vi "Main v0.5.vi"() -> ()   [LabVIEW 2017]
doc: "v0.5:\n\n- Added Reject to Manual Mode\n- Send reject pallet cluster during manual mode\n- Run continuous manual happens only when no error has occured"
uses:
  Controls/Main Tabs.ctl
  Controls/Auto.ctl
  RT/Controls/Auto Delays.ctl
  RT/Controls/Auto Times.ctl
  <userlib>/SESL Controls/refresh ES.ctl
  Controls/UI Data.ctl
  support/Message Queue/Enqueue Message (Single).vi
  <vilib>/Utility/error.llb/Error Cluster From Error Code.vi
  <vilib>/ErrorRing/Error Ring.xnode
  support/Message Queue/Message Queue.lvlib
  support/User Event - Stop/User Event - Stop.lvlib
panel:
  out "Date-Time":string caption="Dip-Tube Assembly Automation (HMI) v0.5"
  out "Main Tab":T1
  in  "Autocycle":T2
  in  "Manual":bool
  in  "Parameters":bool
  in  "Maintenance":bool
  in  "Save Para":bool
  in  "Home Para":bool
  in  "ParaTab":T3(tab)
  in  "StopperRearDelay":dbl format="%#.2f"
  in  "StopperFrontDelay":dbl format="%#.2f"
  in  "MaxAlarms":dbl caption="Max Alarms in 1 Minute" format="%#.2f"
  in  "MaxConsecutive":dbl caption="Max Consecutive Alarms" format="%#.2f"
  in  "Gate Close Delay":dbl format="%#.2f"
  in  "Gate Open Delay":dbl format="%#.2f"
  in  "BF Off Delay":dbl format="%#.2f"
  in  "BF On Delay":dbl format="%#.2f"
  in  "DelayAfterReject":dbl format="%#.2f"
  in  "MeasurementTime":dbl format="%#.2f"
  in  "DelayAfterMesFront":dbl format="%#.2f"
  in  "DelayAfterCut":dbl format="%#.2f"
  in  "DelayAfterCutClamp":dbl format="%#.2f"
  in  "DelayAfterInsClamp":dbl format="%#.2f"
  in  "DelayToClose":dbl format="%#.2f"
  in  "DelayToOpen":dbl format="%#.2f"
  in  "DelayAfterInsertion":dbl format="%#.2f"
  in  "DelayBeforeInsertion":dbl format="%#.2f"
  in  "AgitatorUpTime":dbl format="%#.2f"
  in  "AgitatorDownTime":dbl format="%#.2f"
  in  "Reject Pallets":T4
  in  "Enable Reject?":bool
  in  "Toggle Motor":bool
  in  "Continuous?":T5
  in  "Enable Measure?":bool
  in  "Enable Index?":bool
  in  "Enable PF?":bool
  in  "Auto Delays":T6={"Agitator Delays"=[400], "TF Delays"=[500], "Insertion Delays"=[100, 500], "Cutting Delays"=[150, 500, 100], "PF Delays"=[100], "Measur. Delays"=[500], "Reject Delays"=[500]}
  in  "Enable Cutting?":bool
  in  "Enable Insertion?":bool
  in  "Run Manual":bool
  in  "Enable TF?":bool
  in  "Home Manual":bool
  out "Status":T8
  out "Measurements":T9 {"Height 1" format="%#.2f"; "Height 2" format="%#.2f"; "Height 3" format="%#.2f"; "Height 4" format="%#.2f"}
  out "OutputCount":u32
  in  "All IO":bool
  in  "Stats":bool
  in  "Home AC":bool
  out "Status":string
  out "Count":dbl format="%06.0f"
  out "Count 3":dbl caption="Cycle Time" format="%0.2f"
  out "Count 2":dbl caption="Rejects" format="%06.0f"
  in  "Statuses":string[][](table)
  in  "Exit":bool
  # "Vision Harmony Dip-Tube Assembly Automation"
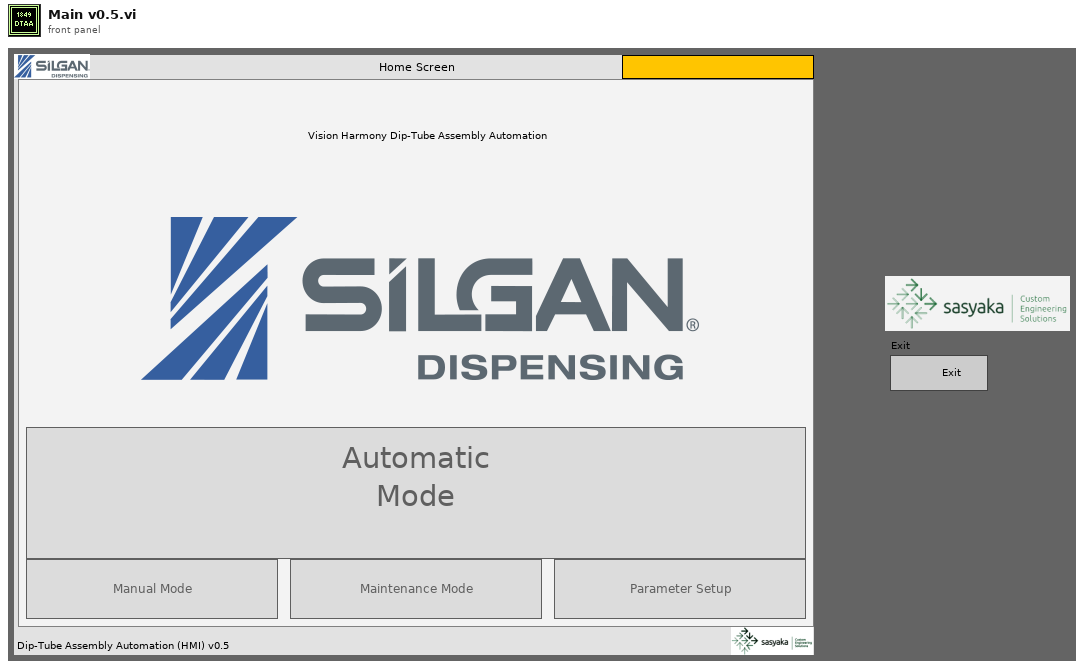
[diagram p1: front panel]
types:
  T1 = typedef "Main Tabs.ctl" = enum32{"Home Screen", "Parameter Setup", "Manual Mode", "Autocycle"}
  T2 = typedef "Auto.ctl" = bool
  T3 = enum32{"General & Indexing", "Bowl Feeder & Pump Conveyor", "Cutting, Measurement & Rejection", "Tube Feeder & Insertion"}
  T4 = cluster{"Reject 1":bool, "Reject 2":bool, "Reject 3":bool, "Reject 4":bool}
  T5 = typedef "refresh ES.ctl" = bool
  T6 = typedef "Auto Delays.ctl" = cluster{"Agitator Delays":u32[], "TF Delays":u32[], "Insertion Delays":u32[], "Cutting Delays":u32[], "PF Delays":u32[], "Measur. Delays":u32[], "Reject Delays":u32[]}
  T7 = typedef "Auto Times.ctl" = cluster{"Index Time":u32, "TF Time":u32, "Insertion Time":u32, "Cutting Time":u32, "PF Time":u32, "Meas. Time":u32, "Reject Time":u32}
  T8 = cluster{"Auto Times":T7, "error out":errorcluster}
  T9 = cluster{"Height 1":dbl, "Height 2":dbl, "Height 3":dbl, "Height 4":dbl}
  T10 = typedef "UI Data.ctl" = cluster{"Main Tab":refnum<vi>}
  T11 = typedef "Message Queue.lvlib/All Message Queues.ctl" = cluster{"UI":refnum<queue>}
  T12 = enum8{"Enabled", "Disabled", "Disabled and Grayed Out"}
  T13 = cluster{"Auto Times":T7, "Measurements":cluster{"1":dbl, "2":dbl, "3":dbl, "4":dbl}, "OutputCount":u32, "error out":errorcluster}
  T14 = cluster{"Auto Delays":T6, "Reject Pallets":cluster{"Reject 1":bool, "Reject 2":bool, "Reject 3":bool, "Reject 4":bool}}
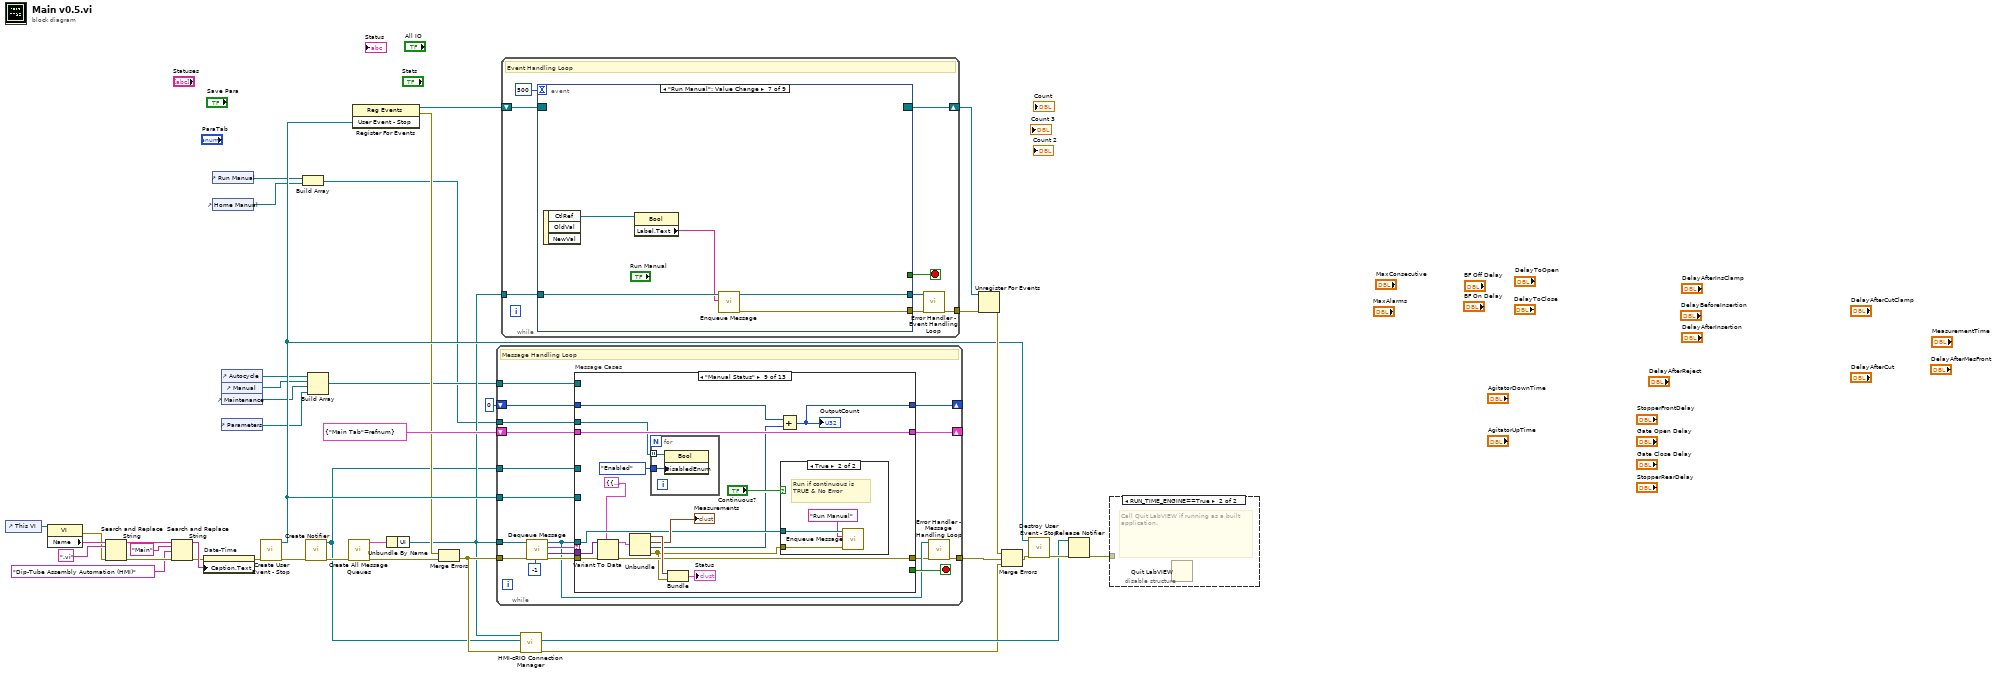
[diagram p0: block diagram]
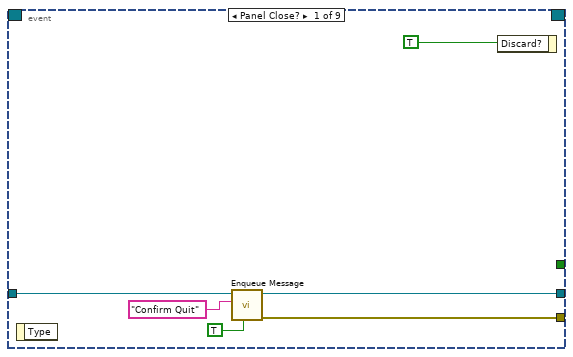
[diagram p2: hidden frame]
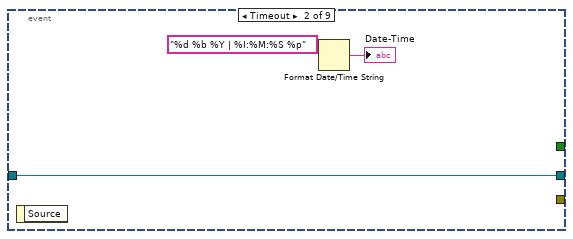
[diagram p3: hidden frame]
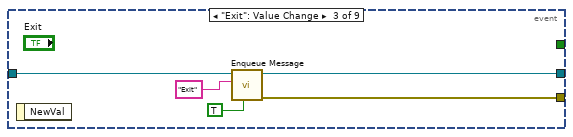
[diagram p4: hidden frame]
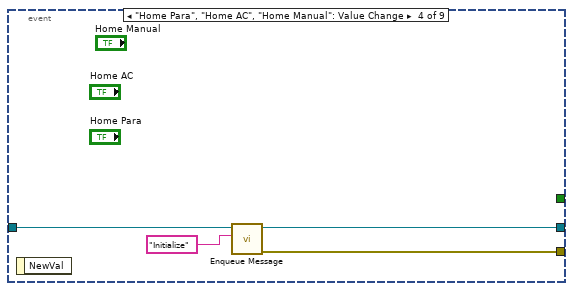
[diagram p5: hidden frame]
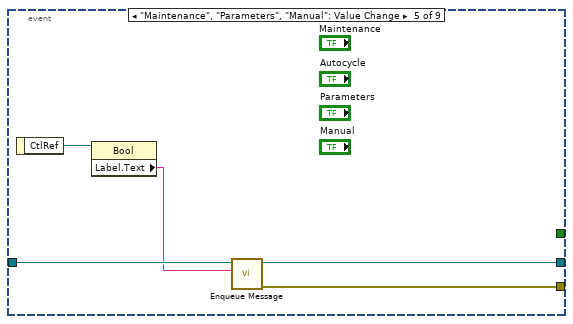
[diagram p6: hidden frame]
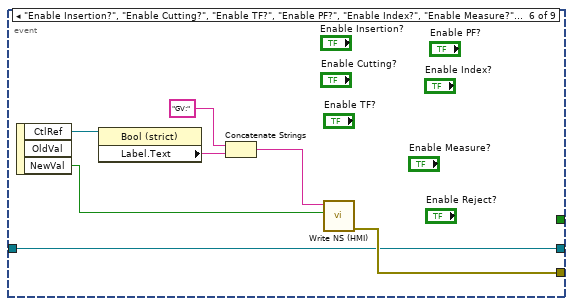
[diagram p7: hidden frame]
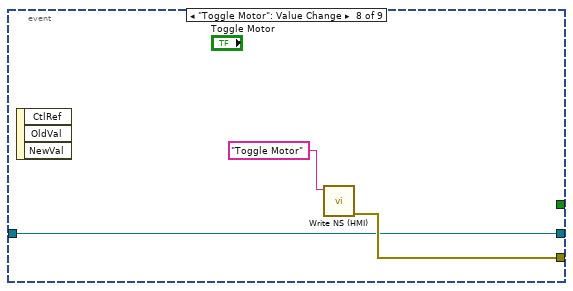
[diagram p8: hidden frame]
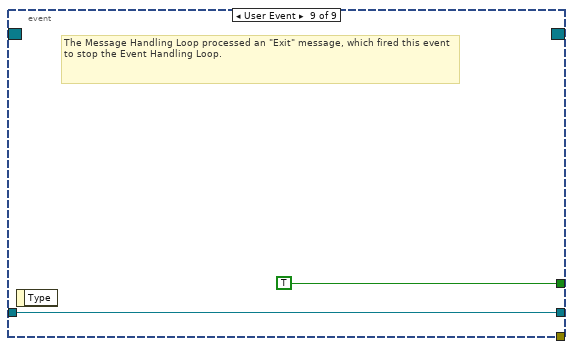
[diagram p9: hidden frame]
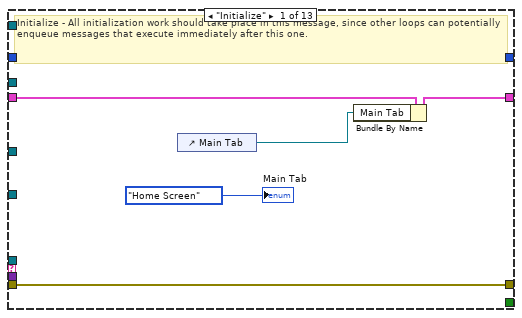
[diagram p10: hidden frame]
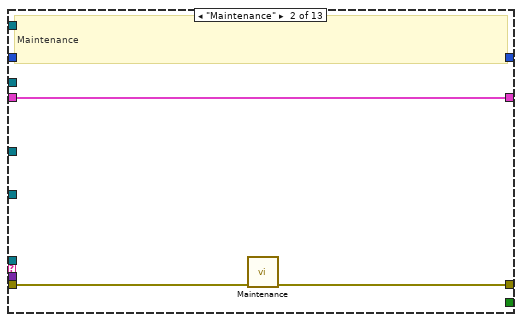
[diagram p11: hidden frame]
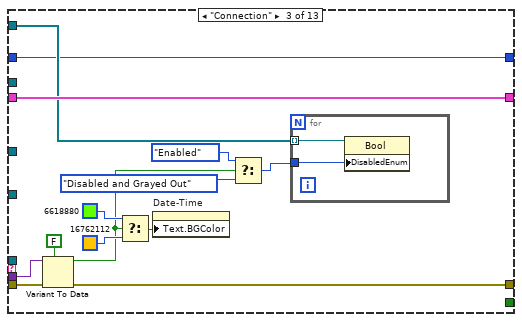
[diagram p12: hidden frame]
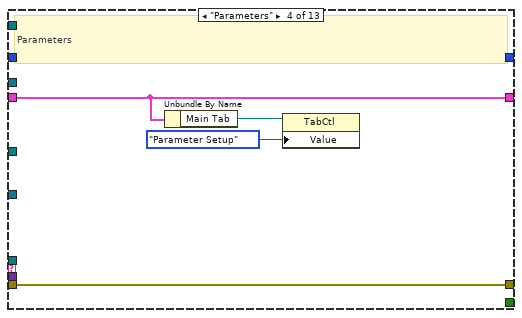
[diagram p13: hidden frame]
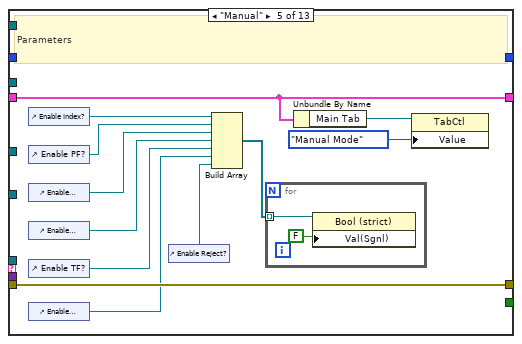
[diagram p14: hidden frame]
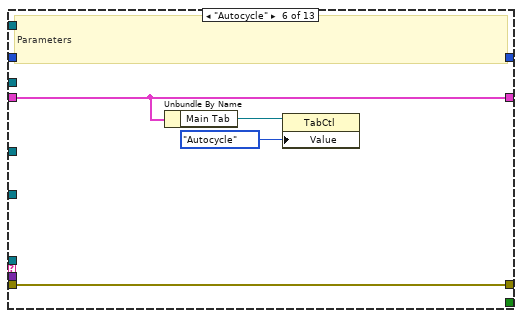
[diagram p15: hidden frame]
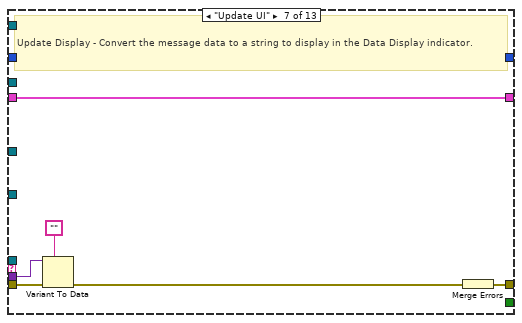
[diagram p16: hidden frame]
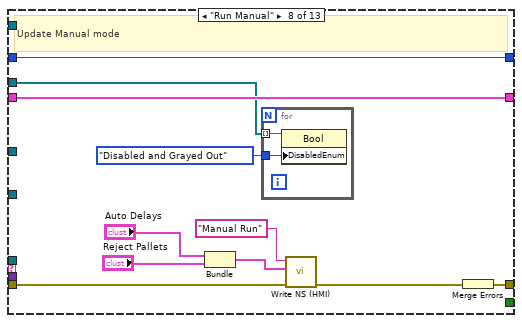
[diagram p17: hidden frame]
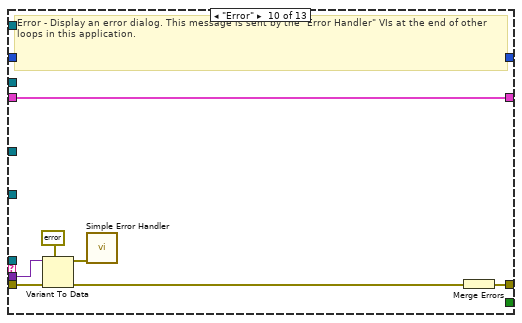
[diagram p19: hidden frame]
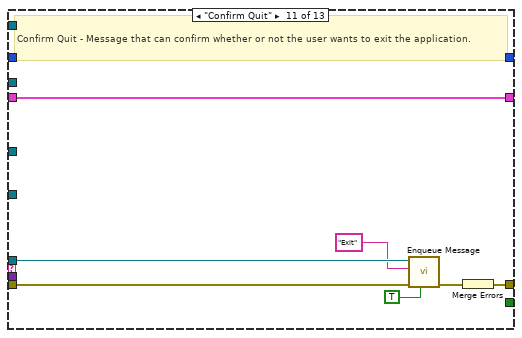
[diagram p20: hidden frame]
diagram:
  n1 = control-ref of="This VI"() -> (w9:refnum<vi>)
  n2 = property class="VI"(reference=w9) -> (error out=w8:errorcluster, "Name"=w15:string)  [unwired: 1 in, 1 out]
  n3 = Search and Replace String(input string=w15, search string=".vi", error in=w8) -> (result string=w13:string, error out=w12:errorcluster)  [unwired: 5 in, 2 out]
  n4 = Search and Replace String(input string=w13, search string="Main", replace string="Dip-Tube Assembly Automation (HMI)" ("replace string (\"\")"), error in=w12) -> (result string=w7:string, error out=w6:errorcluster)  [unwired: 4 in, 2 out]
  n5 = property on="Date-Time" class="Str"(error in=w6, "Caption.Text"=w7) -> (error out=w5:errorcluster)  [unwired: 1 in, 1 out]
  n6 = control-ref of="Run Manual"() -> (w4:refnum<vi>)
  n7 = control-ref of="Home Manual"() -> (w3:refnum<vi>)
  n8 = control-ref of="Autocycle"() -> (w20:refnum<vi>)
  n9 = control-ref of="Manual"() -> (w19:refnum<vi>)
  n10 = control-ref of="Maintenance"() -> (w18:refnum<vi>)
  n11 = control-ref of="Parameters"() -> (w17:refnum<vi>)
  n12 = call "Create User Event - Stop.vi"("error in (no error)"=w5) -> ("error out"=w27:errorcluster, "User Event - Stop"=w31:refnum<user-event>)  [unwired: 9 in]
  n13 = Build Array(w4, w3) -> (w2:refnum<vi>[])
  n14 = call "Create Notifier.vi"("error in (no error)"=w27) -> ("error out"=w26:errorcluster, "notifier out"=w21:refnum<notifier>)  [unwired: 9 in]
  n15 = Build Array(w20, w19, w18, w17) -> (w16:refnum<vi>[])
  n16 = call "Create All Message Queues.vi"("error in (no error)"=w26) -> ("error out"=w40:errorcluster, "Message Queues out"=w39:T11)  [unwired: 9 in]
  n17 = register-events(w31) -> (reference out=w32:refnum<event-registration>, error out=w30:errorcluster)  [unwired: 2 in]
  n18 = Unbundle By Name(w39) -> ("UI"=w28:refnum<queue>)
  n19 = Merge Errors(w30, w40) -> (w29:errorcluster)
  n20 = while {
    tunnel: w28 -> [w50]
    shift-right: [w57] -> _
    shift-left: T10 {"Main Tab"=refnum} ("Data Cluster") -> [w58]
    tunnel: w31 -> [w55]
    tunnel: w29 -> [w54]
    tunnel: [w48] -> w38
    tunnel: w21 -> [w45]
    tunnel: w16 -> [w44]
    tunnel: w2 -> [w43]
    shift-right: [w41] -> _
    shift-left: u32 0 ("OutputCount") -> [w42]
    stop <- w56 stop-if-true
    # "Message Handling Loop"
    n21 = call "Dequeue Message.vi"("timeout"=-1, "error in (no error)"=w54, "Message Queue"=w50) -> ("error out"=w53:errorcluster, "Message Data"=w51:variant, "Message"=w52:string, "dup Message Queue"=w49:refnum<queue>)  [unwired: 5 in]
    n22 = case "Message Cases" shown="\"Manual Status\"" w52 {
      selector: w52 -> [_ _ _ _ _ _ _ _ _ _ _ _ w184]
      tunnel: w49 -> [_ _ _ _ _ _ _ _ w136 _ w163 w182 _]
      tunnel: w53 -> [w64 w67 w80 w89 w102 w109 w114 w124 w145 w159 w167 w175 _]
      tunnel: [w64 w66 w79 w89 w102 w109 w115 w126 w135 w153 w165 w178 w185] -> w47
      tunnel: w58 -> [w63 w68 w82 w88 w101 w108 w116 w127 w146 w158 w166 w181 w186]
      tunnel: [w62 w68 w82 w88 w101 w108 w116 w127 w146 w158 w166 w181 w186] -> w57
      tunnel: [_ _ _ _ _ _ _ _ _ _ _ TRUE _] -> w56
      tunnel: w51 -> [_ _ w78 _ _ _ w113 _ w144 w157 _ w172 _]
      tunnel: w55 -> [_ _ _ _ _ _ _ _ _ _ _ w177 _]
      tunnel: w45 -> [_ _ _ _ _ _ _ _ _ _ _ w171 _]
      tunnel: w44 -> [_ _ w74 _ _ _ _ _ _ _ _ _ _]
      tunnel: w43 -> [_ _ _ _ _ _ _ w121 w142 _ _ _ _]
      tunnel: w42 -> [w59 w65 w69 w85 w90 w105 w110 w117 w132 w152 w160 w168 w183]
      tunnel: [w59 w65 w69 w85 w90 w105 w110 w117 w131 w152 w160 w168 w183] -> w41
      frame "Initialize" {
        # "Initialize - All initialization work should take place in this message, since other loops can potentially enqueue messages that execute immediately after this one."
        n23 = control-ref of="Main Tab"() -> (w61:refnum<vi>)
        n24 = Bundle By Name(cluster=w63, "Main Tab"=w61) -> (w62:T10)
        "Main Tab" <- Main_Tabs."Home Screen" ("Main Tab")
      }
      frame "Maintenance" {
        # "Maintenance"
        n25 = call "Maintenance.vi"("Error In"=w67) -> ("Error out"=w66:errorcluster)  [unwired: 10 in]
      }
      frame "Connection" {
        n26 = Variant To Data(error in=w80, type=FALSE, Variant=w78) -> (data=w73:bool, error out=w79:errorcluster)
        n27 = Select(t=u32 6618880 ("Text.Text Colors:BG Color"), s=w73, f=u32 16762112 ("Text.Text Colors:BG Color")) -> (s? t:f=w75:u32)
        n28 = property on="Date-Time" class="Str"("Text.BGColor"=w75) -> ()  [unwired: 2 in, 2 out]
        n29 = Select(t=T12."Enabled" ("Disabled"), s=w73, f=T12."Disabled and Grayed Out") -> (s? t:f=w71:T12)
        n30 = for {
          tunnel: w74 -> [w84] mode=indexing
          tunnel: w71 -> [w83]
          n31 = property class="Bool"(reference=w84, "DisabledEnum"=w83) -> ()  [unwired: 1 in, 2 out]
        }
      }
      frame "Parameters" {
        # "Parameters"
        n32 = Unbundle By Name(w88) -> ("Main Tab"=w87:refnum<vi>)
        n33 = property class="TabCtl"(reference=w87, "Value"=Main_Tabs."Parameter Setup" ("Main Tab")) -> ()  [unwired: 1 in, 2 out]
      }
      frame "Manual" {
        # "Parameters"
        n34 = control-ref of="Enable Index?"() -> (w98:refnum<vi>)
        n35 = control-ref of="Enable PF?"() -> (w97:refnum<vi>)
        n36 = control-ref of="Enable Cutting?"() -> (w96:refnum<vi>)
        n37 = control-ref of="Enable Insertion?"() -> (w95:refnum<vi>)
        n38 = control-ref of="Enable TF?"() -> (w94:refnum<vi>)
        n39 = control-ref of="Enable Measure?"() -> (w92:refnum<vi>)
        n40 = control-ref of="Enable Reject?"() -> (w91:refnum<vi>)
        n41 = Build Array(w98, w97, w96, w95, w94, w92, w91) -> (w93:refnum<vi>[])
        n42 = for {
          tunnel: w93 -> [w104] mode=indexing
          n43 = property class="Bool (strict)"(reference=w104, "Val(Sgnl)"=FALSE ("Value (Signaling)")) -> ()  [unwired: 1 in, 2 out]
        }
        n44 = Unbundle By Name(w101) -> ("Main Tab"=w100:refnum<vi>)
        n45 = property class="TabCtl"(reference=w100, "Value"=Main_Tabs."Manual Mode" ("Main Tab")) -> ()  [unwired: 1 in, 2 out]
      }
      frame "Autocycle" {
        # "Parameters"
        n46 = Unbundle By Name(w108) -> ("Main Tab"=w107:refnum<vi>)
        n47 = property class="TabCtl"(reference=w107, "Value"=Main_Tabs."Autocycle" ("Main Tab")) -> ()  [unwired: 1 in, 2 out]
      }
      frame "Update UI" {
        # "Update Display - Convert the message data to a string to display in the Data Display indicator."
        n48 = Variant To Data(error in=w114, type="", Variant=w113) -> (error out=w111:errorcluster)  [unwired: 1 out]
        n49 = Merge Errors(w111) -> (w115:errorcluster)
      }
      frame "Run Manual" {
        # "Update Manual mode"
        n50 = Bundle("Auto Delays"="Auto Delays", "Reject Pallets"="Reject Pallets") -> (w118:T14)  [unwired: 1 in]
        n51 = for {
          tunnel: w121 -> [w129] mode=indexing
          tunnel: T12."Disabled and Grayed Out" ("Disabled") -> [w128]
          n52 = property class="Bool"(reference=w129, "DisabledEnum"=w128) -> ()  [unwired: 1 in, 2 out]
        }
        n53 = call "Write NS (HMI).vi"("error in (no error)"=w124, "Message Data"=w118, "Message"="Manual Run") -> ("error out"=w123:errorcluster)  [unwired: 8 in]
        n54 = Merge Errors(w123) -> (w126:errorcluster)
      }
      frame "Manual Status" {
        n55 = Variant To Data(error in=w145, type=T13 {"Auto Times"={"Index Time"=0, "TF Time"=0, "Insertion Time"=0, "Cutting Time"=0, "PF Time"=0, "Meas. Time"=0, "Reject Time"=0}, "Measurements"={"1"=0.0, "2"=0.0, "3"=0.0, "4"=0.0}, "OutputCount"=0, "error out"={"status"=FALSE, "code"=0, "source"=""}} ("cluster"), Variant=w144) -> (data=w141:T13, error out=w135:errorcluster)
        n56 = Unbundle(w141) -> ("Auto Times"=w140:T7, "Measurements"=→"Measurements":cluster{"1":dbl, "2":dbl, "3":dbl, "4":dbl}, "OutputCount"=w133:u32, "error out"=w130:errorcluster)
        n57 = for {
          tunnel: w142 -> [w151] mode=indexing
          tunnel: T12."Enabled" ("Disabled") -> [w150]
          n58 = property class="Bool"(reference=w151, "DisabledEnum"=w150) -> ()  [unwired: 1 in, 2 out]
        }
        n59 = Bundle("Auto Times"=w140, "error out"=w130) -> (→"Status":T8)  [unwired: 1 in]
        n60 = Add(x=w132, y=w133) -> (x+y=w131:u32)
        "OutputCount" <- w131
        n61 = case shown="True" "Continuous?" {
          tunnel: w136 -> [_ w149]
          tunnel: w130 -> [_ w148]
          frame False {
          }
          frame True {
            # "Run if continuous is TRUE & No Error"
            n62 = call-poly "Enqueue Message.vi"("error in (no error)"=w148, "Message"="Run Manual", "Message Queue"=w149) -> ()  [unwired: 7 in, 2 out]
          }
        }
      }
      frame "Error" {
        # "Error - Display an error dialog. This message is sent by the \"Error Handler\" VIs at the end of other loops in this application."
        n63 = Variant To Data(error in=w159, type=errorcluster {"status"=FALSE, "code"=0, "source"=""} ("error constant"), Variant=w157) -> (data=w155:errorcluster, error out=w154:errorcluster)
        n64 = call <vilib>:"Simple Error Handler.vi"("error in (no error)"=w155) -> ()  [unwired: 4 in, 5 out]
        n65 = Merge Errors(w154) -> (w153:errorcluster)
      }
      frame "Confirm Quit" {
        # "Confirm Quit - Message that can confirm whether or not the user wants to exit the application."
        n66 = call-poly "Enqueue Message.vi"("Priority Message? (F)"=TRUE, "error in (no error)"=w167, "Message"="Exit", "Message Queue"=w163) -> ("error out"=w164:errorcluster)  [unwired: 6 in, 1 out]
        n67 = Merge Errors(w164) -> (w165:errorcluster)
      }
      frame "Exit" {
        # "Stop the VI"
        # "Release the message queue reference"
        # "Exit - Exit the application."
        n68 = Variant To Data(type=errorcluster {"status"=FALSE, "code"=0, "source"=""} ("error constant"), Variant=w172) -> (data=w173:errorcluster)  [unwired: 1 in, 1 out]
        n69 = call <vilib>:"Simple Error Handler.vi"("error in (no error)"=w173) -> ()  [unwired: 4 in, 5 out]
        n70 = Send Notification(notification=TRUE, notifier=w171) -> (error out=w169:errorcluster)  [unwired: 1 in, 1 out]
        n71 = call "Fire User Event - Stop.vi"("User Event - Stop"=w177) -> ("error out"=w176:errorcluster)  [unwired: 10 in]
        n72 = Release Queue(queue=w182, error in (no error)=w175) -> (error out=w179:errorcluster)  [unwired: 1 in, 2 out]
        n73 = Merge Errors(w169, w176, w179) -> (w178:errorcluster)
      }
      frame Default {
        # "'Default' case only runs if there is a message that isn't defined in any of the other cases.  Output a programming error."
        n74 = xnode "Error Ring"("parameter 0"=w184) -> ("error out"=w185:errorcluster)
      }
    }
    n75 = call "Error Handler - Message Handling Loop.vi"("error in (no error)"=w47, "Message Queue"=w49) -> ("dup error in"=w48:errorcluster)  [unwired: 8 in, 1 out]
  }
  n76 = while {
    tunnel: w28 -> [w201]
    shift-right: [w199] -> w35
    shift-left: w32 -> [w200]
    tunnel: [w195] -> w33
    stop <- w197 stop-if-true
    # "Event Handling Loop"
    n77 = event shown="[6] \"Run Manual\": Value Change" {
      selector: w200 -> [_ _ _ _ _ _ _ _ _]
      dyn-events: [_ _ _ _ _ _ _ _ _] -> w199
      timeout: 500 -> [_ _ _ _ _ _ _ _ _]
      tunnel: [_ _ _ _ _ _ _ _ TRUE ("Discard?")] -> w197
      tunnel: w201 -> [w206 w210 w215 w219 w224 w229 w236 w238 w241]
      tunnel: [w205 _ w214 w218 w223 w230 w234 w239 _] -> w198
      tunnel: [w204 w210 w213 w217 w222 w229 w235 w238 w241] -> w196
      event Panel Close? {
        n78 = event-data() -> ()  [unwired: 1 in, 1 out]
        n79 = call-poly "Enqueue Message.vi"("Priority Message? (F)"=TRUE, "Message"="Confirm Quit", "Message Queue"=w206) -> ("error out"=w205:errorcluster, "dup Message Queue"=w204:refnum<queue>)  [unwired: 7 in]
        n80 = event-data("Discard?"=TRUE) -> ()  [unwired: 1 in, 1 out]
      }
      event Timeout {
        n81 = event-data() -> ()  [unwired: 1 in, 1 out]
        n82 = Format Date/Time String(time format string (%c)="%d %b %Y | %I:%M:%S %p") -> (date/time string=→"Date-Time":string)  [unwired: 2 in]
      }
      event "Exit": Value Change {
        n83 = event-data() -> ()  [unwired: 1 in, 1 out]
        n84 = call-poly "Enqueue Message.vi"("Priority Message? (F)"=TRUE, "Message"="Exit", "Message Queue"=w215) -> ("error out"=w214:errorcluster, "dup Message Queue"=w213:refnum<queue>)  [unwired: 7 in]
      }
      event "Home Para", "Home AC", "Home Manual": Value Change {
        n85 = event-data() -> ()  [unwired: 1 in, 1 out]
        n86 = call-poly "Enqueue Message.vi"("Message"="Initialize", "Message Queue"=w219) -> ("error out"=w218:errorcluster, "dup Message Queue"=w217:refnum<queue>)  [unwired: 8 in]
      }
      event "Maintenance", "Parameters", "Manual": Value Change {
        n87 = event-data() -> ("CtlRef"=w221:refnum<vi>)  [unwired: 1 in]
        n88 = property class="Bool"(reference=w221) -> ("Label.Text"=w220:string)  [unwired: 1 in, 2 out]
        n89 = call-poly "Enqueue Message.vi"("Message"=w220, "Message Queue"=w224) -> ("error out"=w223:errorcluster, "dup Message Queue"=w222:refnum<queue>)  [unwired: 8 in]
      }
      event "Enable Insertion?", "Enable Cutting?", "Enable TF?", "Enable PF?", "Enable Index?", "Enable Measure?", "Enable Reject?": Value Change {
        n90 = event-data() -> ("CtlRef"=w231:refnum<vi>, "NewVal"=w225:bool)  [unwired: 1 in, 1 out]
        n91 = property class="Bool (strict)"(reference=w231) -> ("Label.Text"=w228:string)  [unwired: 1 in, 2 out]
        n92 = Concatenate Strings("GV:" ("string"), w228) -> (w226:string)
        n93 = call "Write NS (HMI).vi"("Message Data"=w225, "Message"=w226) -> ("error out"=w230:errorcluster)  [unwired: 9 in]
      }
      event "Run Manual": Value Change {
        n94 = event-data() -> ("CtlRef"=w233:refnum<vi>)  [unwired: 1 in, 2 out]
        n95 = property class="Bool"(reference=w233) -> ("Label.Text"=w232:string)  [unwired: 1 in, 2 out]
        n96 = call-poly "Enqueue Message.vi"("Message"=w232, "Message Queue"=w236) -> ("error out"=w234:errorcluster, "dup Message Queue"=w235:refnum<queue>)  [unwired: 8 in]
      }
      event "Toggle Motor": Value Change {
        n97 = event-data() -> ()  [unwired: 1 in, 3 out]
        n98 = call "Write NS (HMI).vi"("Message"="Toggle Motor") -> ("error out"=w239:errorcluster)  [unwired: 10 in]
      }
      event User Event {
        # "The Message Handling Loop processed an \"Exit\" message, which fired this event to stop the Event Handling Loop."
        n99 = event-data() -> ()  [unwired: 1 in, 1 out]
      }
    }
    n100 = call "Error Handler - Event Handling Loop.vi"("error in (no error)"=w198, "Message Queue"=w196) -> ("dup error in"=w195:errorcluster)  [unwired: 8 in, 1 out]
  }
  n101 = call "HMI-cRIO Connection Manager.vi"("error in"=w29, "notifier in"=w21, "Queue in"=w28) -> ("error out"=w22:errorcluster, "Notifier out"=w23:refnum<notifier>)  [unwired: 7 in]
  n102 = Unregister For Events(event registration refnum=w35, error in=w33) -> (error out=w36:errorcluster)
  n103 = Merge Errors(w36, w38, w22) -> (w37:errorcluster)
  n104 = call "Destroy User Event - Stop.vi"("error in (no error)"=w37, "User Event - Stop"=w31) -> ("error out"=w25:errorcluster)  [unwired: 9 in]
  n105 = Release Notifier(notifier=w23, error in (no error)=w25) -> (error out=w24:errorcluster)  [unwired: 1 in, 2 out]
  n106 = disable-structure shown="RUN_TIME_ENGINE==True" {
    disable-tunnel: w24 -> [_ _]
    frame condition #0 (active) {
    }
    frame condition #1 {
      # "Call Quit LabVIEW if running as a built application."
      n107 = Quit LabVIEW() -> ()  [unwired: 1 in]
    }
  }
